vi "T7MOD_Write_FLOAT32_Register.vi"(7 "FLOAT32 to Write":sgl=1.23, 8 "error in":errorcluster, 9 "LabJack FLOAT32 Register":i32=55124, 10 "Remote Port":u16=502, 11 "Remote IP Address":string="192.168.1.15") -> (0 "error out":errorcluster, 1 "Written At":timestamp)   [LabVIEW 2018]
panel:
  # "Input"
  # "TCP Parameters"
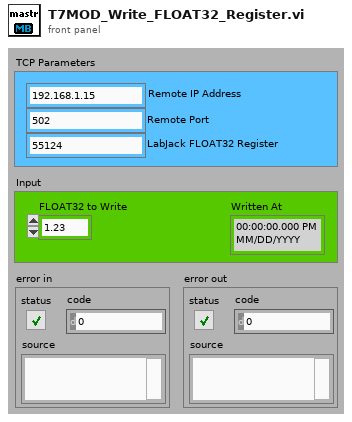
[diagram p1: front panel]
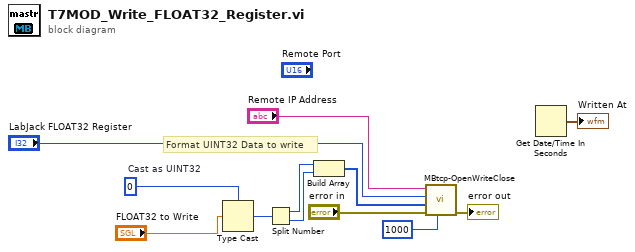
[diagram p0: block diagram]
diagram:
  w11 = u32 0  # Cast as UINT32
  # "Format UINT32 Data to write"
  n1 = Type Cast(type=w11, x="FLOAT32 to Write") -> (*(type *) &x=w10:u32)
  n2 = Split Number(x=w10) -> (hi(x)=w9:u16, lo(x)=w8:u16)
  n3 = Build Array(w9, w8) -> (w4:u16[])
  n4 = call "MBtcp-OpenWriteClose.vi"("Timeout (900)"=1000 ("timeout ms (60000)"), "error in (no error)"="error in", "Values"=w4, "RegisterAddr"="LabJack FLOAT32 Register", "IP Address(:port)"="Remote IP Address") -> ("error out"=→"error out":errorcluster)  [unwired: 6 in]
  n5 = Get Date/Time In Seconds() -> (seconds since 1Jan1904=→"Written At":timestamp)
